vi "Tulip handler.vi"(6 "Table ID":string="d96D6nKvoPkdenefz", 7 "State":T2(ring), 8 "error in":errorcluster, 9 "Body":T1, 10 "Authentication":cluster{"Username":string, "Password":string}={"Username"="apikey.2_WNWgDzkcRL7LwQrSC", "Password"="uUTRYqQF2kxie-OG2NdFiDN_Ok5rwnamrdCqWvd0OVz"}, 11 "URL":string="https://outset-medical-staging.tulip.co/") -> (0 "error out":errorcluster, 1 "Status String":string, 2 "Response body":string)   [LabVIEW 2021]
uses:
  <vilib>/addons/_JKI.lib/REST Client/classes/REST Client/REST Client.lvclass
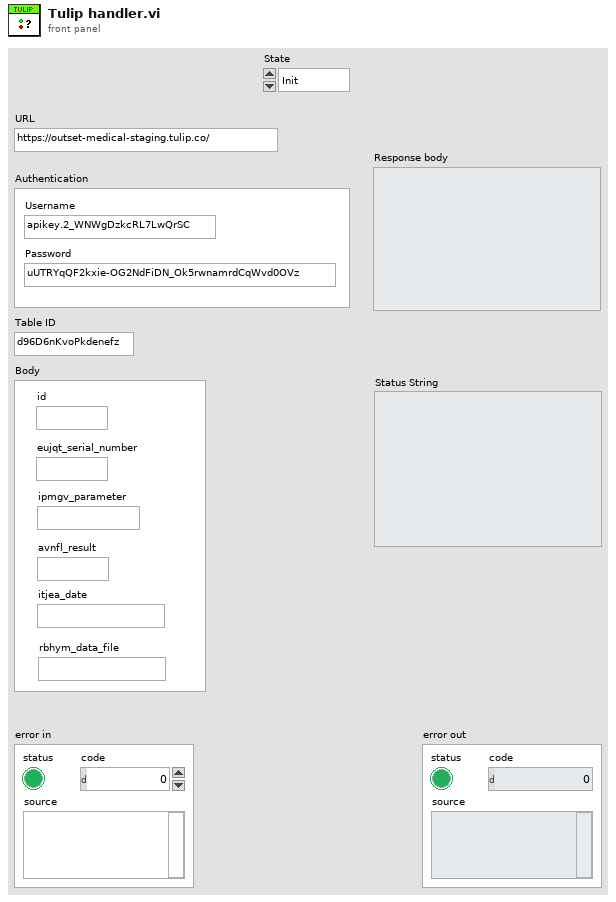
[diagram p1: front panel]
types:
  T1 = cluster{"id":string, "eujqt_serial_number":string, "ipmgv_parameter":string, "avnfl_result":string, "itjea_date":string, "rbhym_data_file":string}
  T2 = enum16{"Init", "Get headers", "Get", "Post", "Put", "Close"}
  T3 = typedef "REST Client.lvlib/REST Client.lvclass/HTTP Header.ctl" = cluster{"header":string, "value":string}
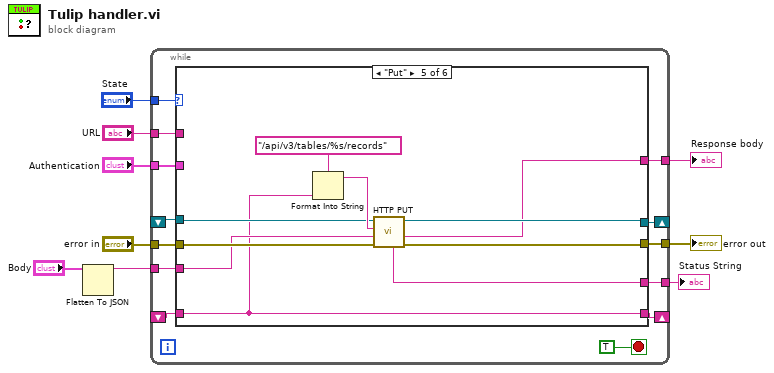
[diagram p0: block diagram]
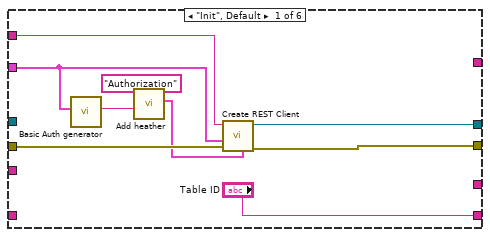
[diagram p2: hidden frame]
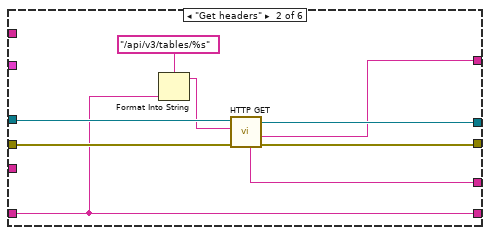
[diagram p3: hidden frame]
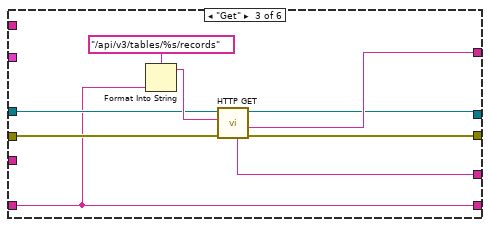
[diagram p4: hidden frame]
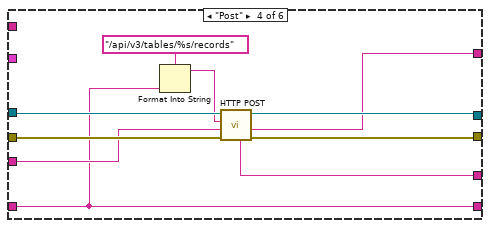
[diagram p5: hidden frame]
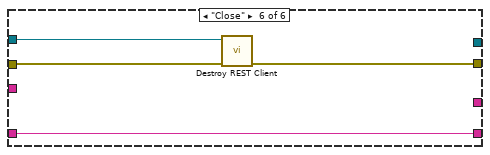
[diagram p6: hidden frame]
diagram:
  n1 = Flatten To JSON(anything="Body") -> (JSON string=w2:string)  [unwired: 2 in, 1 out]
  n2 = while {
    tunnel: "State" -> [w21]
    tunnel: "URL" -> [w20]
    shift-right: [w19] -> _
    shift-left: _ -> [w14]
    tunnel: "Authentication" -> [w18]
    tunnel: "error in" -> [w17]
    tunnel: [w16] -> w5
    tunnel: [w13] -> w4
    tunnel: w2 -> [w12]
    shift-right: [w11] -> _
    shift-left: _ -> [w15]
    tunnel: [w10] -> w1
    stop <- TRUE stop-if-true
    n3 = case shown="\"Put\"" w21 {
      tunnel: w20 -> [w31 _ _ _ _ _]
      tunnel: [w30 w37 w43 w56 w65 _] -> w19
      tunnel: w18 -> [w27 _ _ _ _ _]
      tunnel: w17 -> [w29 w40 w49 w59 w68 w73]
      tunnel: [w28 w38 w48 w58 w64 w72] -> w16
      tunnel: w15 -> [_ w35 w42 w51 w62 w70]
      tunnel: w14 -> [_ w39 w45 w57 w66 w71]
      tunnel: [_ w36 w44 w52 w63 _] -> w13
      tunnel: w12 -> [_ _ _ w53 w67 _]
      tunnel: ["Table ID" w35 w42 w51 w62 w70] -> w11
      tunnel: [_ w34 w41 w50 w60 _] -> w10
      frame "Init", Default {
        n4 = call "Basic Auth generator.vi"("Authentication"=w27) -> ("Basic Auth"=w25:string)  [unwired: 10 in]
        n5 = call "Add heather.vi"("value"=w25, "header"="Authorization") -> ("headers"=w24:T3[])  [unwired: 9 in]
        n6 = call <vilib>:"Create REST Client.vi"("Default Headers ([JSON])"=w24, "error in (no error)"=w29, "Authentication"=w27, "Base URL"=w31) -> ("error out"=w28:errorcluster, "REST Client out"=w30:refnum<class "REST Client.lvclass">)  [unwired: 6 in]
      }
      frame "Get headers" {
        n7 = Format Into String(format string="/api/v3/tables/%s", w35) -> (resulting string=w33:string)  [unwired: 2 in, 1 out]
        n8 = call-dynamic "HTTP GET.vi"("error in (no error)"=w40, "Path"=w33, "REST Client in"=w39) -> ("error out"=w38:errorcluster, "Response body"=w36:string, "REST Client out"=w37:refnum<class "REST Client.lvclass">, "Status String"=w34:string)  [unwired: 3 in, 2 out]
      }
      frame "Get" {
        n9 = Format Into String(format string="/api/v3/tables/%s/records", w42) -> (resulting string=w47:string)  [unwired: 2 in, 1 out]
        n10 = call-dynamic "HTTP GET.vi"("error in (no error)"=w49, "Path"=w47, "REST Client in"=w45) -> ("error out"=w48:errorcluster, "Response body"=w44:string, "REST Client out"=w43:refnum<class "REST Client.lvclass">, "Status String"=w41:string)  [unwired: 3 in, 2 out]
      }
      frame "Post" {
        n11 = Format Into String(format string="/api/v3/tables/%s/records", w51) -> (resulting string=w54:string)  [unwired: 2 in, 1 out]
        n12 = call-dynamic "HTTP POST.vi"("error in (no error)"=w59, "Request body"=w53, "Path"=w54, "REST Client in"=w57) -> ("error out"=w58:errorcluster, "Response body"=w52:string, "REST Client out"=w56:refnum<class "REST Client.lvclass">, "Status String"=w50:string)  [unwired: 2 in, 2 out]
      }
      frame "Put" {
        n13 = Format Into String(format string="/api/v3/tables/%s/records", w62) -> (resulting string=w69:string)  [unwired: 2 in, 1 out]
        n14 = call-dynamic "HTTP PUT.vi"("error in (no error)"=w68, "Request body"=w67, "Path"=w69, "REST Client in"=w66) -> ("error out"=w64:errorcluster, "Response body"=w63:string, "REST Client out"=w65:refnum<class "REST Client.lvclass">, "Status String"=w60:string)  [unwired: 2 in, 2 out]
      }
      frame "Close" {
        n15 = call-dynamic "Destroy REST Client.vi"("error in (no error)"=w73, "REST Client in"=w71) -> ("error out"=w72:errorcluster)  [unwired: 9 in]
      }
    }
  }
  "error out" <- w5
  "Response body" <- w4
  "Status String" <- w1
